vi "fip-trigger.vi"() -> ()   [LabVIEW 2022 SP3]
doc: "I. Description:\nThis example demonstrates how to continuously output a waveform using an internal sample clock. The automatic regeneration of data has been disabled, so new data has to be provided throughout the duration of the continuous Analog Output operation. This allows the generation of any arbitrary frequency as this VI computes new data for each iteration of the loop, maintaining phase continuity of the signal.\n\nII. Instructions for Running:\n1. Select the Physical Channel to correspond to where your signal is output on the DAQ device.\n2. Enter the Minimum and Maximum Voltage range.\n3. Specify the desired Sample Clock Rate of the output Waveform. Higher sample clock rates will produce a smoother waveform.\n4. Manually specify the Analog Output buffer size, in number of samples. A larger buffer would help non-regenerative operations avoid errors due to occasional high CPU load. \nNote: \nThe Analog Output buffer has to be at least as big as the amount of data being written to the board per iteration. The recommended buffer size would be at least twice the amount of data being written to the board per iteration.\n5. Enter the Waveform Information. See the documentation of the Basic Function Generator SubVI for information on each parameter.\n\nIII. Block Diagram Steps:\n1. Create an Analog Output Voltage channel.\n2. Configure the task to prohibit the automatic regeneration of data.\n3. Call the DAQmx (Sample Clock) VI to set the sample clock rate. Additionally, set the sample mode to Continuous.\n4. Read the actual sample clock rate (eventually coerced depending on the hardware used). \n5. Compute the desired waveform, using the buffer size and the actual update rate. This VI keeps track of the phase of the waveform to ensure that the generated signal is continuous.\n6. Write the waveform to the output buffer. \n7a. Call the Start VI. This is only needed when the loop is executed for the first time.\n7b. Do nothing.\n8. Loop continuously until user presses the Stop button. Every iteration computes and writes a new waveform to the buffer.\n9. Call the Clear Task VI to clear the Task.\n10. Use the popup dialog box to display an error or warning if any.\n\nIV. I/O Connections Overview:\nMake sure your signal output terminal matches the Physical Channel I/O Control. For further connection information, refer to your hardware reference manual."
uses:
  <vilib>/Utility/error.llb/DialogType.ctl
  <vilib>/DAQmx/write.llb/DAQmx Write (Analog 1D Wfm NChan NSamp).vi
  <vilib>/DAQmx/create/channels.llb/DAQmx Create Channel (AO-Voltage-Basic).vi
  <vilib>/DAQmx/configure/timing.llb/DAQmx Timing (Sample Clock).vi
  <vilib>/DAQmx/miscellaneous.llb/DAQmx Fill In Error Info.vi
  <vilib>/measure/NI_MABase.lvlib
  <resource>/objmgr/daqmx.rc
panel:
  in  "Offset 1":dbl=2.5
  in  "Offset 3":dbl=2.5
  in  "Offset 2":dbl=2.5
  in  "Offset 4":dbl=2.5
  in  "Phase 4":dbl=120.0
  in  "Duty Cycle 4":dbl=30.0
  in  "Duty Cycle 3":dbl=30.0
  in  "Duty Cycle 2":dbl=30.0
  in  "Duty Clycle 1":dbl=50.0
  in  "Phase 2":dbl
  in  "Phase 3":dbl=240.0
  in  "Phase 1":dbl=-70.0
  in  "Amplitude 1":dbl=2.5 caption="Amplitude" format="%0.2p"
  in  "Frequency 1":dbl=27.0 caption="Frequency" format="%.2f"
  in  "Waveform Type 1":T1(ring)=enum."Square Wave" caption="Waveform Type"
  in  "CH 1 ON":bool=TRUE
  in  "Amplitude 2":dbl=2.5 caption="Amplitude" format="%0.2p"
  in  "Frequency 2":dbl=9.0 caption="Frequency" format="%.2f"
  in  "Waveform Type 2":T1(ring)=enum."Square Wave" caption="Waveform Type"
  in  "CH 2 ON":bool=TRUE
  in  "CH 4 ON":bool=TRUE
  in  "CH 3 ON":bool=TRUE
  in  "Waveform Type 3":T1(ring)=enum."Square Wave" caption="Waveform Type"
  in  "Frequency 3":dbl=9.0 caption="Frequency" format="%.2f"
  in  "Amplitude 3":dbl=2.5 caption="Amplitude" format="%0.2p"
  in  "Waveform Type 4":T1(ring)=enum."Square Wave" caption="Waveform Type"
  in  "Frequency 4":dbl=9.0 caption="Frequency" format="%.2f"
  in  "Amplitude 4":dbl=2.5 caption="Amplitude" format="%0.2p"
  in  "Size (Samples)":u32=20000
  out "Actual Sample Clock Rate":dbl=20000.0 format="%.2f"
  in  "Sample Clock Rate":dbl=20000.0 format="%0.2f"
  out "Waveform Graph":waveform(dbl)[](graph)=[{"t0"=timestamp(7.25 s since 1904-01-01), "dt"=5e-05, "Y"=array[5000 elements]}, {"t0"=timestamp(7.25 s since 1904-01-01), "dt"=5e-05, "Y"=array[5000 elements]}] caption="Output Waveform"
  in  "Physical Channels":tag="Dev1/ao0:3"
  in  "Minimum Value":dbl=-10.0 format="%0.2f"
  in  "Maximum Value":dbl=10.0 format="%0.2f"
  in  "stop":bool
  # "For instructions, select Help>>Show Context Help"
  # "Channel Parameters"
  # "Timing Parameters"
  # "Waveform Information"
  # "Buffer Parameters"
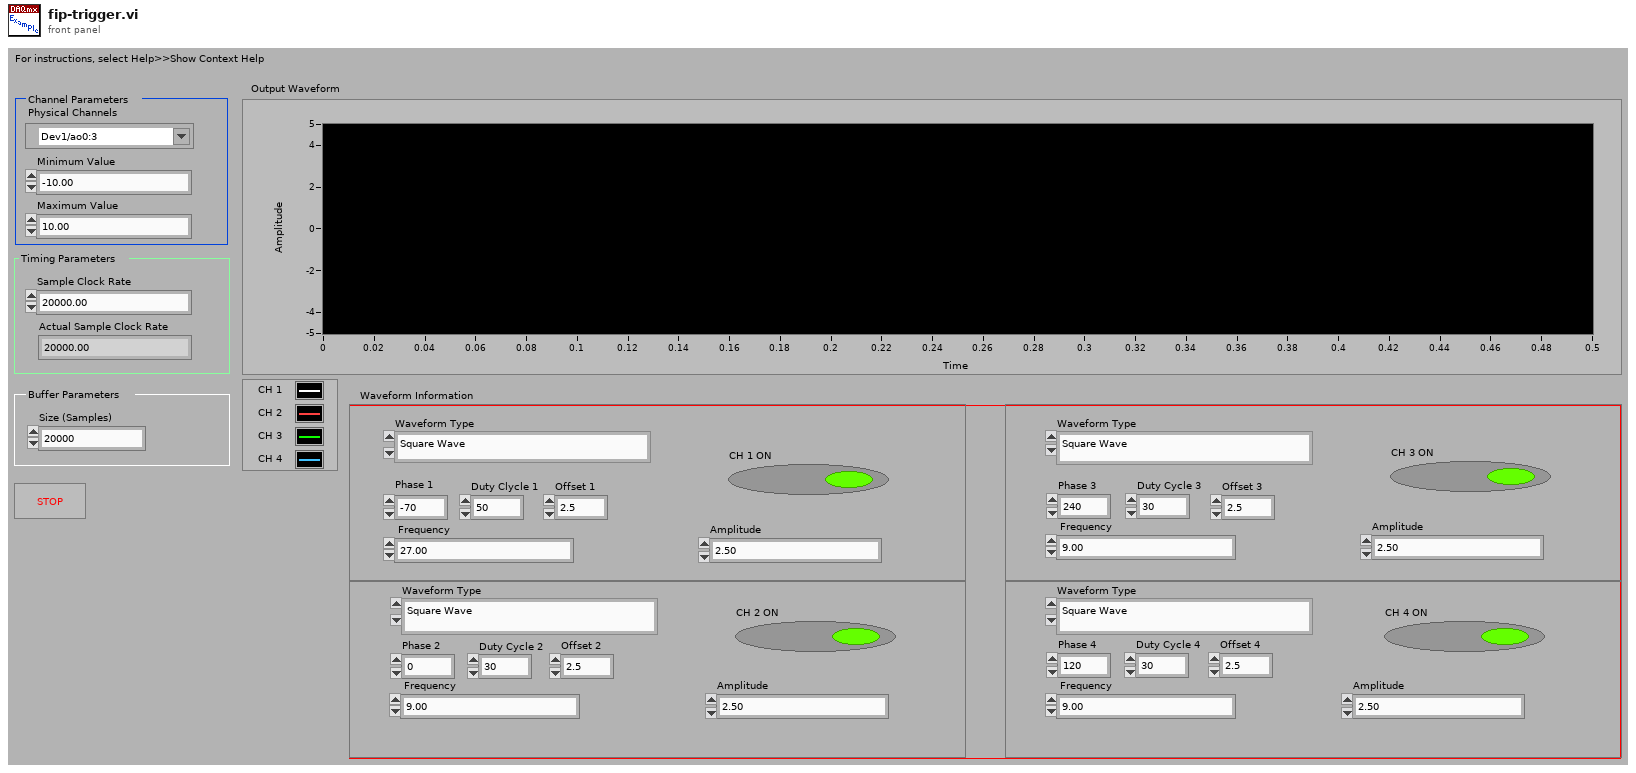
[diagram p1: front panel]
types:
  T1 = enum16{"Sine Wave", "Triangle Wave", "Square Wave", "Sawtooth Wave"}
  T2 = typedef "DialogType.ctl" = u16
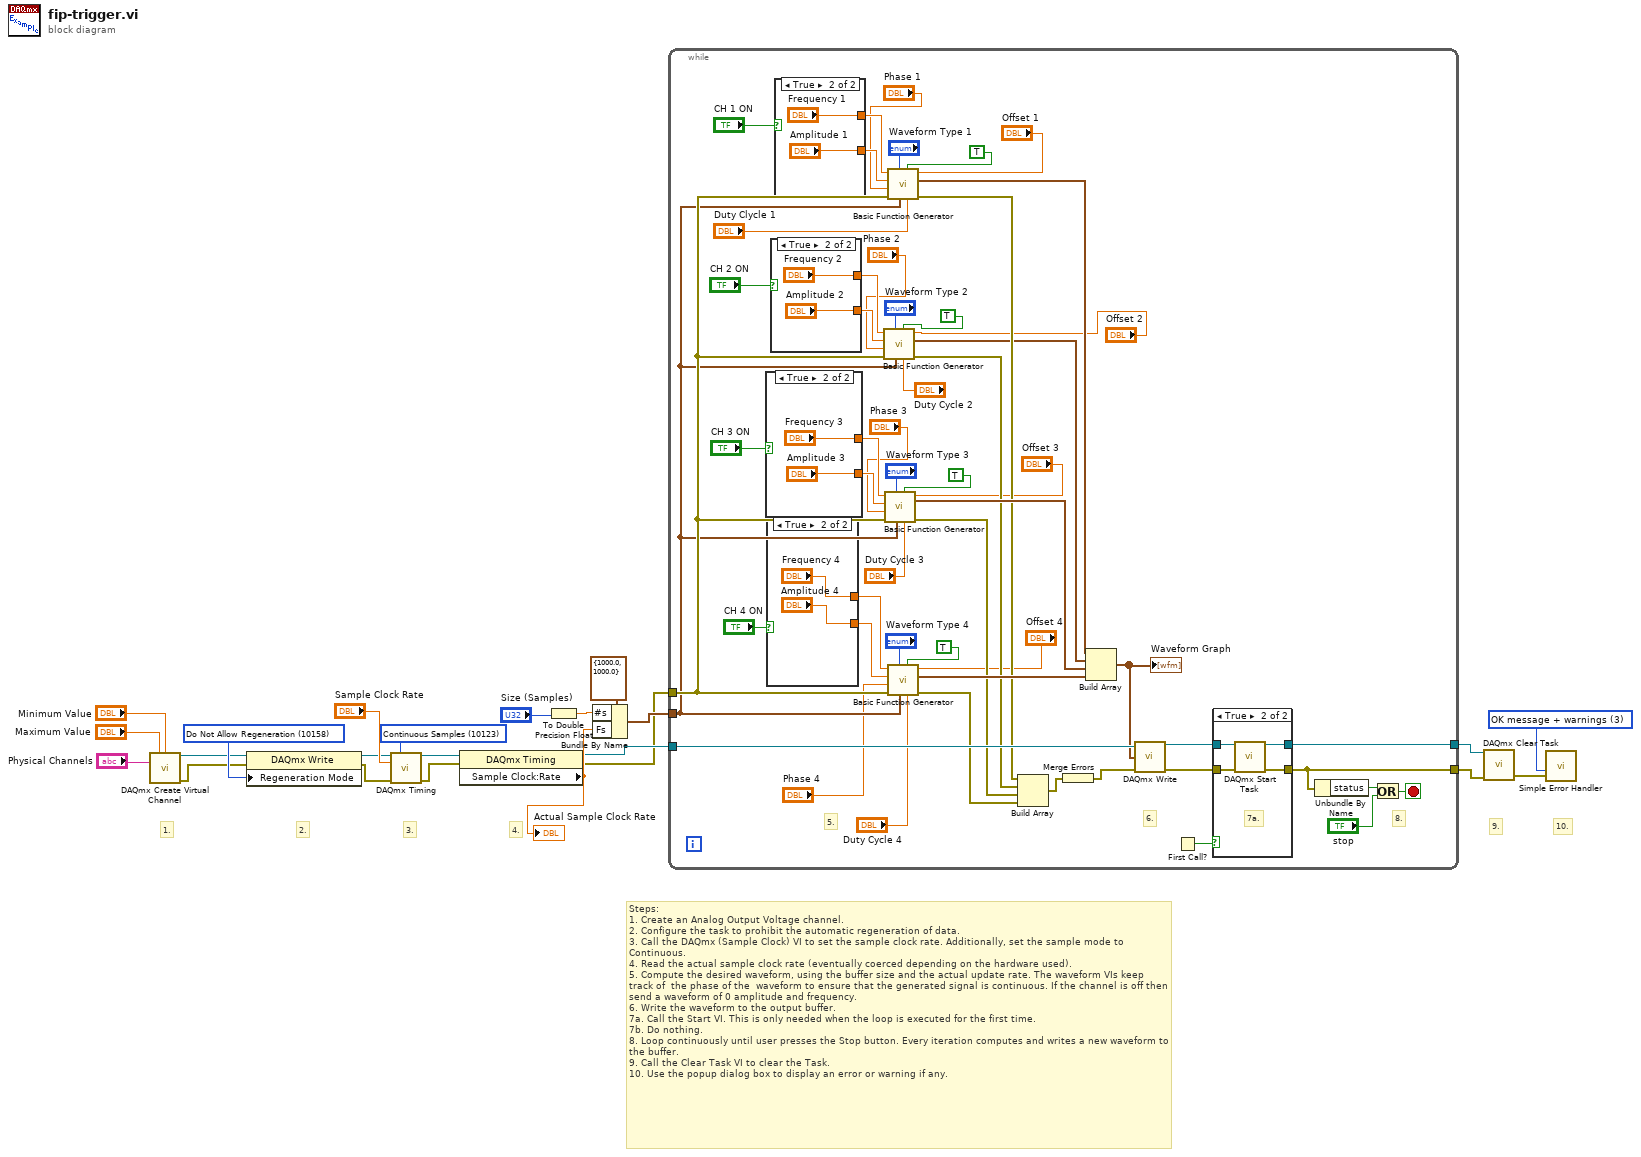
[diagram p0: block diagram]
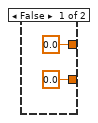
[diagram p2: hidden frame]
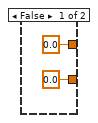
[diagram p3: hidden frame]
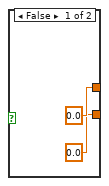
[diagram p4: hidden frame]
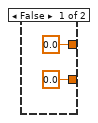
[diagram p5: hidden frame]
diagram:
  w12 = 10158 items=["Allow Regeneration"=10097, "Do Not Allow Regeneration"=10158] ("RegenMode")
  w21 = T2 3 items=["no dialog", "OK message", "continue or stop message", "OK message + warnings", "continue/stop + warnings"] ("type of dialog (OK msg:1)")
  w22 = 10123 items=["Finite Samples"=10178, "Continuous Samples"=10123] ("sample mode")
  # "4."
  # "3."
  # "Steps:\n1. Create an Analog Output Voltage channel.\n2. Configure the task to prohibit the automatic regeneration of data.\n3. Call the DAQmx (Sample Clock) VI to set the sample clock rate. Additionally, set the sample mode to Continuous.\n4. Read the actual sample clock rate (eventually coerced depending on the hardware used).\n5. Compute the desired waveform, using the buffer size and the actual update rate. The waveform VIs keep track of  the phase of the  waveform to ensure that the generated signal is continuous. If the channel is off then send a waveform of 0 amplitude and frequency.\n6. Write the waveform to the output buffer. \n7a. Call the Start VI. This is only needed when the loop is executed for the first time.\n7b. Do nothing.\n8. Loop continuously until user presses the Stop button. Every iteration computes and writes a new waveform to the buffer.\n9. Call the Clear Task VI to clear the Task.\n10. Use the popup dialog box to display an error or warning if any."
  # "10."
  # "9."
  # "2."
  # "1."
  n1 = call-poly <vilib>:"DAQmx Create Virtual Channel.vi"("maximum value"="Maximum Value", "minimum value"="Minimum Value", "physical channels"="Physical Channels") -> ("task out"=w2:refnum<k21>, "error out"=w1:errorcluster)  [unwired: 6 in, 5 out]
  n2 = property class="DAQmx Write"(reference=w2, error in=w1, "Regeneration Mode"=w12) -> (reference out=w7:refnum<k21>, error out=w6:errorcluster)
  n3 = call-poly <vilib>:"DAQmx Timing.vi"("task/channels in"=w7, "sample mode"=w22, "rate"="Sample Clock Rate", "error in"=w6) -> ("task out"=w17:refnum<k21>, "error out"=w16:errorcluster)  [unwired: 3 in, 7 out]
  n4 = property class="DAQmx Timing"(reference=w17, error in=w16) -> (reference out=w11:refnum<k21>, error out=w10:errorcluster, "Sample Clock:Rate"=w14:dbl)
  "Actual Sample Clock Rate" <- w14
  n5 = To Double Precision Float(number="Size (Samples)") -> (double precision float=w8:dbl)
  n6 = Bundle By Name(cluster=cluster{"Fs":dbl, "#s":dbl} {"Fs"=1000.0, "#s"=1000.0} ("sampling info"), "#s"=w8, "Fs"=w14) -> (w13:cluster{"Fs":dbl, "#s":dbl})
  n7 = while {
    tunnel: w11 -> [w74]
    tunnel: [w70] -> w20
    tunnel: w10 -> [w48]
    tunnel: [w71] -> w19
    tunnel: w13 -> [w47]
    stop <- w77 stop-if-true
    # "8."
    # "6."
    # "5."
    n8 = case shown="True" "CH 3 ON" {
      tunnel: [0.0 ("Amplitude 2") "Amplitude 3"] -> w64
      tunnel: [0.0 ("Frequency 2") "Frequency 3"] -> w63
      frame False {
      }
      frame True {
      }
    }
    n9 = case shown="True" "CH 4 ON" {
      tunnel: [0.0 ("Amplitude") "Amplitude 4"] -> w61
      tunnel: [0.0 ("Frequency") "Frequency 4"] -> w60
      frame False {
      }
      frame True {
      }
    }
    n10 = case shown="True" "CH 2 ON" {
      tunnel: [0.0 ("Amplitude 2") "Amplitude 2"] -> w56
      tunnel: [0.0 ("Frequency 2") "Frequency 2"] -> w55
      frame False {
      }
      frame True {
      }
    }
    n11 = case shown="True" "CH 1 ON" {
      tunnel: [0.0 ("Amplitude 2") "Amplitude 1"] -> w52
      tunnel: [0.0 ("Frequency 2") "Frequency 1"] -> w51
      frame False {
      }
      frame True {
      }
    }
    n12 = call <vilib>:"Basic Function Generator.vi"("offset"="Offset 2", "square wave duty cycle (%)"="Duty Cycle 2", "reset signal"=TRUE, "sampling info"=w47, "signal type"="Waveform Type 2", "error in (no error)"=w48, "phase"="Phase 2", "amplitude"=w56, "frequency"=w55) -> ("error out"=w43:errorcluster, "signal out"=w45:waveform(dbl))  [unwired: 1 out]
    n13 = call <vilib>:"Basic Function Generator.vi"("offset"="Offset 3", "square wave duty cycle (%)"="Duty Cycle 3", "reset signal"=TRUE, "sampling info"=w47, "signal type"="Waveform Type 3", "error in (no error)"=w48, "phase"="Phase 3", "amplitude"=w64, "frequency"=w63) -> ("error out"=w42:errorcluster, "signal out"=w68:waveform(dbl))  [unwired: 1 out]
    n14 = call <vilib>:"Basic Function Generator.vi"("offset"="Offset 1", "square wave duty cycle (%)"="Duty Clycle 1", "reset signal"=TRUE, "sampling info"=w47, "signal type"="Waveform Type 1", "error in (no error)"=w48, "phase"="Phase 1", "amplitude"=w52, "frequency"=w51) -> ("error out"=w46:errorcluster, "signal out"=w44:waveform(dbl))  [unwired: 1 out]
    n15 = call <vilib>:"Basic Function Generator.vi"("offset"="Offset 4", "square wave duty cycle (%)"="Duty Cycle 4", "reset signal"=TRUE, "sampling info"=w47, "signal type"="Waveform Type 4", "error in (no error)"=w48, "phase"="Phase 4", "amplitude"=w61, "frequency"=w60) -> ("error out"=w41:errorcluster, "signal out"=w67:waveform(dbl))  [unwired: 1 out]
    n16 = Build Array(w46, w43, w42, w41) -> (w40:errorcluster[])
    n17 = Merge Errors(w40) -> (w65:errorcluster)
    n18 = Build Array(w44, w45, w68, w67) -> (w66:waveform(dbl)[])
    "Waveform Graph" <- w66
    n19 = call-poly <vilib>:"DAQmx Write.vi"("task/channels in"=w74, "data"=w66, "error in"=w65) -> ("task out"=w73:refnum<k21>, "error out"=w72:errorcluster)  [unwired: 1 in, 10 out]
    n20 = First Call?() -> (First Call?: T/F=w69:bool)
    n21 = case shown="True" w69 {
      tunnel: w73 -> [w95 w99]
      tunnel: w72 -> [w94 w98]
      tunnel: [w94 w97] -> w71
      tunnel: [w95 w96] -> w70
      frame False {
        # "7b."
      }
      frame True {
        # "7a."
        n22 = call <vilib>:"DAQmx Start Task.vi"("task/channels in"=w99, "error in"=w98) -> ("task out"=w96:refnum<k21>, "error out"=w97:errorcluster)  [unwired: 12 out]
      }
    }
    n23 = Unbundle By Name(w71) -> ("status"=w76:bool)
    n24 = Or(x=w76, y="stop") -> (x .or. y?=w77:bool)
  }
  n25 = call <vilib>:"DAQmx Clear Task.vi"("task in"=w20, "error in"=w19) -> ("error out"=w23:errorcluster)  [unwired: 13 out]
  n26 = call <vilib>:"Simple Error Handler.vi"("type of dialog (OK msg:1)"=w21, "error in (no error)"=w23) -> ()  [unwired: 8 out]
